vi "Bundle Script_Named (Un)Bundler Remove.vi"(4 "Hide Full Names":bool=TRUE, 7 "Change Full Name Visibilty Status":bool=TRUE, 8 "error in":errorcluster, 9 "Selected Item Indices":i32[](array[numeric]), 10 "Selected Items (tags)":string[](array[string]), 11 "Affected Items":T1) -> (0 "error out":errorcluster, 2 "Objects":refnum<vi>[](array[refnum]))   [LabVIEW 2023]
doc: "Takes teg list OR indices list. The latter so we can use this as a subVI easily."
uses:
  top/BundleMagic.ctl
panel:
  # "OR"
  # "HACK! Used to ignore Hide Full Names input"
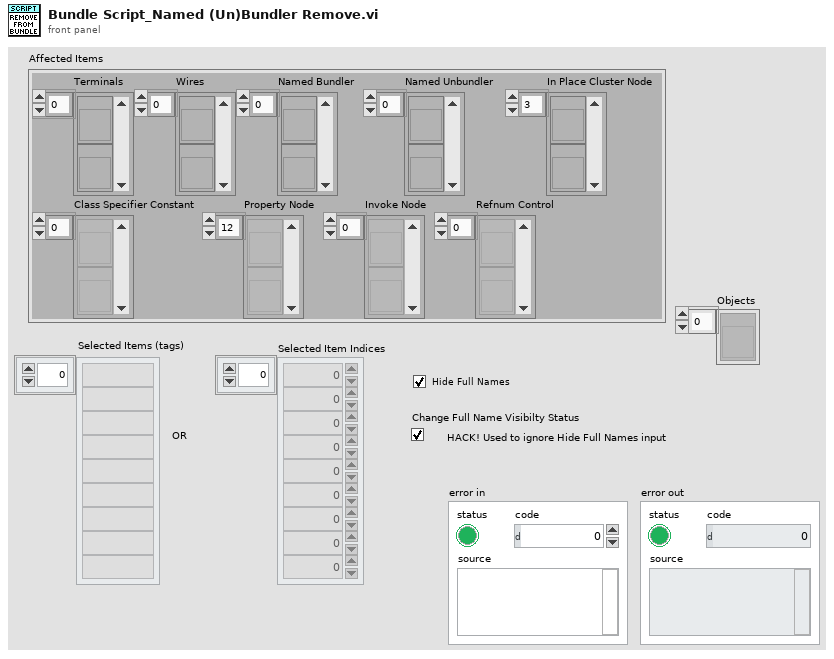
[diagram p1: front panel]
types:
  T1 = typedef "BundleMagic.ctl" = cluster{"Terminals":refnum<vi>[], "Wires":refnum<vi>[], "Named Bundler":refnum<vi>[], "Named Unbundler":refnum<vi>[], "In Place Cluster Node":refnum<vi>[], "Class Specifier Constant":refnum<vi>[], "Property Node":refnum<vi>[], "Invoke Node":refnum<vi>[], "Refnum Control":refnum<vi>[]}
  T2 = enum16{"Named Bundler", "Named Unbundler", "In Place", "None"}
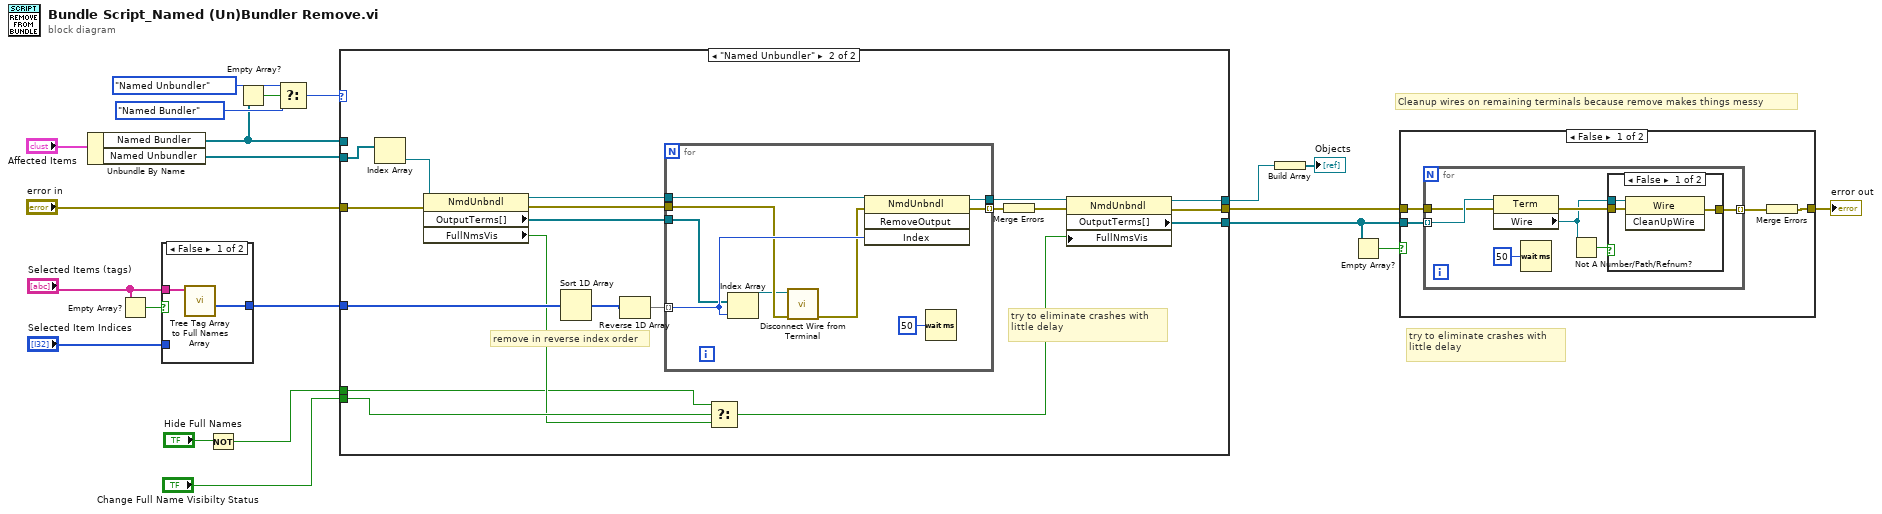
[diagram p0: block diagram]
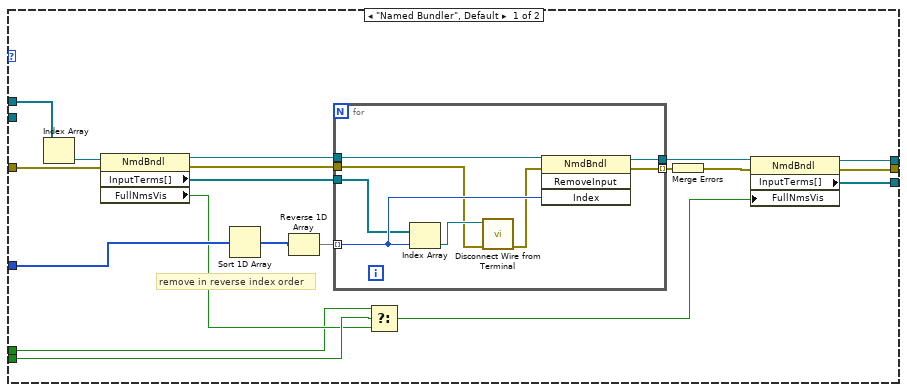
[diagram p5: hidden frame]
diagram:
  # "try to eliminate crashes with little delay"
  # "Cleanup wires on remaining terminals because remove makes things messy"
  n1 = Unbundle By Name("Affected Items") -> ("Named Bundler"=w15:refnum<vi>[], "Named Unbundler"=w14:refnum<vi>[])
  n2 = Empty Array?(array="Selected Items (tags)") -> (empty?=w6:bool)
  n3 = case shown="False" w6 {
    tunnel: "Selected Items (tags)" -> [w23 _]
    tunnel: [w22 w24] -> w12
    tunnel: "Selected Item Indices" -> [_ w24]
    frame False {
      n4 = call "Tree Tag Array to Full Names Array.vi"("Selected Items Tags"=w23) -> ("Selected Item Indices"=w22:u32[])  [unwired: 6 in, 4 out]
    }
    frame True {
    }
  }
  n5 = Not(x="Hide Full Names") -> (.not. x?=w2:bool)
  n6 = Empty Array?(array=w15) -> (empty?=w20:bool)
  n7 = Select(t=T2."Named Unbundler" ("Bundler Type"), s=w20, f=T2."Named Bundler" ("Bundler Type")) -> (s? t:f=w16:T2)
  n8 = case shown="\"Named Unbundler\"" w16 {
    tunnel: [w29 w58] -> w10
    tunnel: "error in" -> [w36 w64]
    tunnel: w15 -> [w35 _]
    tunnel: w14 -> [_ w63]
    tunnel: w12 -> [w34 w62]
    tunnel: [w30 w57] -> w11
    tunnel: [w31 w56] -> w8
    tunnel: w2 -> [w25 w52]
    tunnel: "Change Full Name Visibilty Status" -> [w28 w55]
    frame "Named Bundler", Default {
      # "remove in reverse index order"
      n9 = Index Array(array=w35) -> (element=w37:refnum<vi>)  [unwired: 1 in]
      n10 = property class="NmdBndl"(reference=w37, error in=w36) -> (reference out=w41:refnum<vi>, error out=w40:errorcluster, "InputTerms[]"=w39:refnum<vi>[], "FullNmsVis"=w27:bool)
      n11 = Sort 1D Array(array=w34) -> (sorted array=w43:u32[])
      n12 = Reverse 1D Array(array=w43) -> (reversed array=w42:u32[])
      n13 = for {
        tunnel: w42 -> [w51] mode=indexing
        tunnel: w41 -> [w50]
        tunnel: w40 -> [w45]
        tunnel: w39 -> [w49]
        tunnel: [w48] -> w38 mode=indexing
        tunnel: [w47] -> w32
        n14 = Index Array(array=w49, index=w51) -> (element=w46:refnum<vi>)
        n15 = call "Disconnect Wire from Terminal.vi"("error in"=w45, "Terminal in"=w46) -> ("error out"=w44:errorcluster)  [unwired: 5 in, 4 out]
        n16 = invoke class="NmdBndl" method="RemoveInput"(reference=w50, error in=w44, "Index"=w51) -> (reference out=w47:refnum<vi>, error out=w48:errorcluster)  [unwired: 1 in, 2 out]
      }
      n17 = Select(t=w25, s=w28, f=w27) -> (s? t:f=w26:bool)
      n18 = Merge Errors(w38) -> (w33:errorcluster)
      n19 = property class="NmdBndl"(reference=w32, error in=w33, "FullNmsVis"=w26) -> (reference out=w30:refnum<vi>, error out=w29:errorcluster, "InputTerms[]"=w31:refnum<vi>[])
    }
    frame "Named Unbundler" {
      # "try to eliminate crashes with little delay"
      # "remove in reverse index order"
      n20 = Index Array(array=w63) -> (element=w65:refnum<vi>)  [unwired: 1 in]
      n21 = property class="NmdUnbndl"(reference=w65, error in=w64) -> (reference out=w68:refnum<vi>, error out=w67:errorcluster, "OutputTerms[]"=w61:refnum<vi>[], "FullNmsVis"=w54:bool)
      n22 = Sort 1D Array(array=w62) -> (sorted array=w70:u32[])
      n23 = Reverse 1D Array(array=w70) -> (reversed array=w69:u32[])
      n24 = for {
        tunnel: w69 -> [w79] mode=indexing
        tunnel: w68 -> [w78]
        tunnel: w67 -> [w74]
        tunnel: [w77] -> w66 mode=indexing
        tunnel: w61 -> [w76]
        tunnel: [w75] -> w60
        n25 = Index Array(array=w76, index=w79) -> (element=w72:refnum<vi>)
        n26 = call "Disconnect Wire from Terminal.vi"("error in"=w74, "Terminal in"=w72) -> ("error out"=w73:errorcluster)  [unwired: 5 in, 4 out]
        n27 = invoke class="NmdUnbndl" method="RemoveOutput"(reference=w78, error in=w73, "Index"=w79) -> (reference out=w75:refnum<vi>, error out=w77:errorcluster)  [unwired: 1 in, 2 out]
        n28 = Wait (ms)(milliseconds to wait=u32 50) -> ()  [unwired: 1 out]
      }
      n29 = Select(t=w52, s=w55, f=w54) -> (s? t:f=w53:bool)
      n30 = Merge Errors(w66) -> (w59:errorcluster)
      n31 = property class="NmdUnbndl"(reference=w60, error in=w59, "FullNmsVis"=w53) -> (reference out=w57:refnum<vi>, error out=w58:errorcluster, "OutputTerms[]"=w56:refnum<vi>[])
    }
  }
  n32 = Build Array(w11) -> (→"Objects":refnum<vi>[])
  n33 = Empty Array?(array=w8) -> (empty?=w7:bool)
  n34 = case shown="False" w7 {
    tunnel: w8 -> [w83 _]
    tunnel: w10 -> [w82 w95]
    tunnel: [w80 w95] -> w9
    frame False {
      n35 = for {
        tunnel: w83 -> [w89] mode=indexing
        tunnel: w82 -> [w88]
        tunnel: [w87] -> w81 mode=indexing
        n36 = property class="Term"(reference=w89, error in=w88) -> (error out=w90:errorcluster, "Wire"=w86:refnum<vi>)  [unwired: 1 out]
        n37 = Wait (ms)(milliseconds to wait=u32 50) -> ()  [unwired: 1 out]
        n38 = Not A Number/Path/Refnum?(number/path/refnum=w86) -> (NaN/Path/Refnum?=w85:bool)
        n39 = case shown="False" w85 {
          tunnel: w86 -> [w93 _]
          tunnel: w90 -> [w92 w94]
          tunnel: [w91 w94] -> w87
          frame False {
            n40 = invoke class="Wire" method="CleanUpWire"(reference=w93, error in=w92) -> (error out=w91:errorcluster)  [unwired: 1 in, 2 out]
          }
          frame True {
          }
        }
      }
      n41 = Merge Errors(w81) -> (w80:errorcluster)
    }
    frame True {
    }
  }
  "error out" <- w9
